vi "executeComponentLevelStatemachine.vi"(8 "error in (no error)":errorcluster, 11 "ComponentData in":refnum<class "ComponentData.lvclass">) -> (0 "error out":errorcluster, 3 "ComponentData out":refnum<class "ComponentData.lvclass">)   [LabVIEW 2013, in "ComponentData.lvlib" / "ComponentData.lvclass"]
uses:
  <userlib>/Common/Component/Application/RT/ComponentData/ComponentData/ComponentData.lvclass
  <userlib>/Common/Component/Application/RT/ComponentData/ComponentState/StandbyState/StandbyState.lvclass
  <userlib>/Common/Component/Application/RT/ComponentData/componentStateValues.ctl
  <userlib>/Common/Component/Application/RT/ComponentData/ComponentData/ComponentData.lvclass/ComponentData.ctl
  <userlib>/Common/Component/Application/RT/ComponentData/ComponentState/ComponentState/ComponentState.lvclass
  <userlib>/Common/Component/Application/RT/ComponentData.lvlib
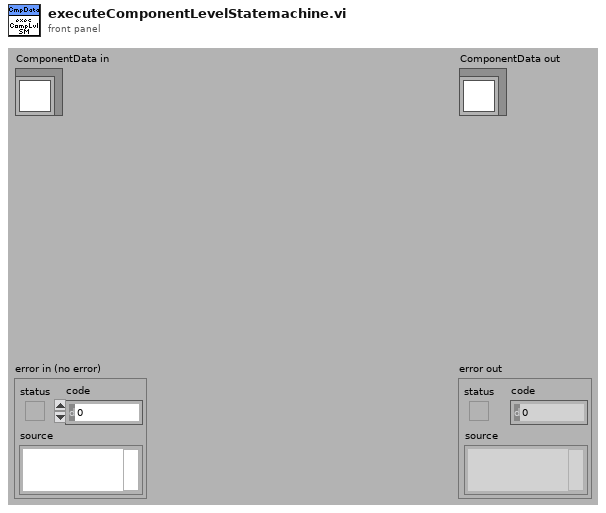
[diagram p1: front panel]
types:
  T1 = typedef "ComponentData.lvlib/componentStateValues.ctl" = enum16{"Off", "Standby", "Enabled", "Disabled", "Fault"}
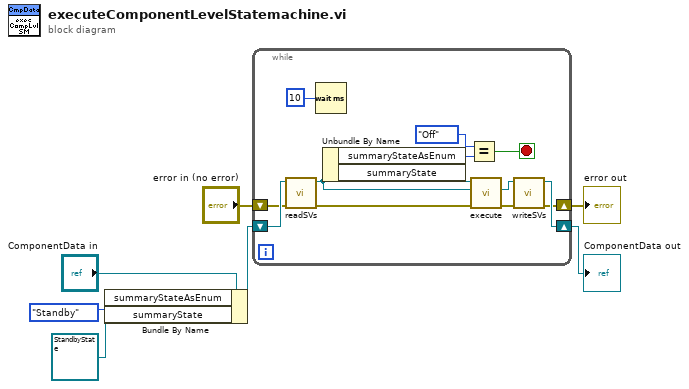
[diagram p0: block diagram]
diagram:
  n1 = Bundle By Name(cluster="ComponentData in", "summaryStateAsEnum"=componentStateValues."Standby", "summaryState"=refnum<class "StandbyState.lvclass"> refnum ("OffState.lvclass")) -> (w1:refnum<class "ComponentData.lvclass">)
  n2 = while {
    shift-right: [w14] -> w5
    shift-left: w1 -> [w11]
    shift-right: [w12] -> w6
    shift-left: "error in (no error)" -> [w9]
    stop <- w17 stop-if-true
    n3 = call-dynamic "readSVs.vi"("error in (no error)"=w9, "ComponentData in"=w11) -> ("error out"=w8:errorcluster, "ComponentData out"=w10:refnum<class "ComponentData.lvclass">)  [unwired: 8 in]
    n4 = Wait (ms)(milliseconds to wait=u32 10) -> ()  [unwired: 1 out]
    n5 = Unbundle By Name(w10) -> ("summaryStateAsEnum"=w19:T1, "summaryState"=w20:refnum<class "ComponentState.lvclass">)
    n6 = Equal?(x=componentStateValues."Off", y=w19) -> (x = y?=w17:bool)
    n7 = call-dynamic "execute.vi"("error in (no error)"=w8, "ComponentData.lvclass"=w10, "ComponentState in"=w20) -> ("error out"=w13:errorcluster, "ComponentData.lvclass 2"=w15:refnum<class "ComponentData.lvclass">)  [unwired: 6 in, 1 out]
    n8 = call-dynamic "writeSVs.vi"("error in (no error)"=w13, "ComponentData in"=w15) -> ("error out"=w12:errorcluster, "ComponentData out"=w14:refnum<class "ComponentData.lvclass">)  [unwired: 8 in]
  }
  "error out" <- w6
  "ComponentData out" <- w5
